vi "extract_pressure_SPT25.vi"(6 "name":string="AIN1", 8 "name_array":string[](array[string]), 9 "value_array":dbl[](array[numeric]), 11 "time":timestamp) -> (0 "P":dbl, 2 "V":dbl, 3 "waveform_array":waveform(dbl)[](array[waveform])=[{"t0"=timestamp(0 s since 1904-01-01), "dt"=1.0, "Y"=[]}, {"t0"=timestamp(3732035173.078092 s since 1904-01-01), "dt"=1.0, "Y"=[302.8589782714844], "attributes"=variant("NI_ChannelName"=variant(string "T1"))}])   [LabVIEW 2019]
panel:
  in  "V_max":dbl=10.0
  in  "V_min":dbl
  in  "P_max":dbl=30.0
  in  "P_min":dbl=-14.7
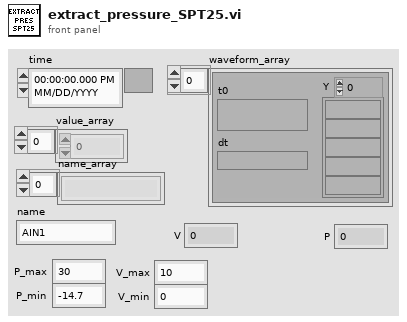
[diagram p1: front panel]
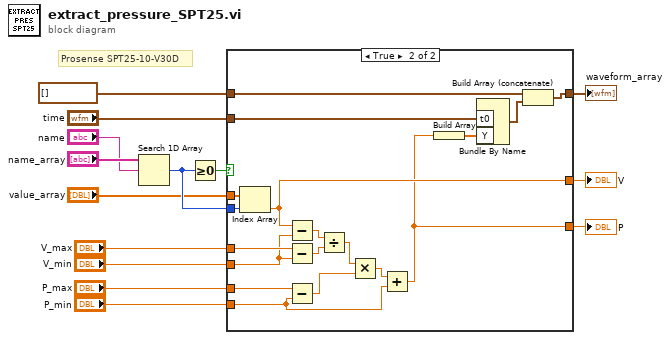
[diagram p0: block diagram]
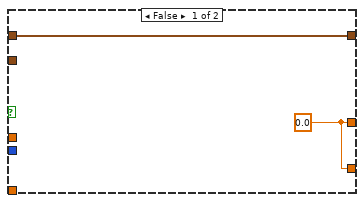
[diagram p2: hidden frame]
diagram:
  # "Prosense SPT25-10-V30D"
  n1 = Search 1D Array(1D array="name_array", element="name") -> (index of element=w11:i32)  [unwired: 1 in]
  n2 = Greater Or Equal To 0?(x=w11) -> (x >= 0?=w12:bool)
  n3 = case shown="True" w12 {
    tunnel: w11 -> [_ w34]
    tunnel: "value_array" -> [_ w33]
    tunnel: waveform(dbl)[] [] -> [w16 w32]
    tunnel: "time" -> [_ w31]
    tunnel: [w16 w30] -> w7
    tunnel: [w15 w17] -> w6
    tunnel: [w15 w25] -> w5
    tunnel: "P_min" -> [_ w18]
    tunnel: "P_max" -> [_ w22]
    tunnel: "V_max" -> [_ w27]
    tunnel: "V_min" -> [_ w26]
    frame False {
      w15 = 0.0 ("CJC (K)")
    }
    frame True {
      n4 = Index Array(array=w33, index=w34) -> (element=w25:dbl)
      n5 = Subtract(x=w25, y=w26) -> (x-y=w23:dbl)
      n6 = Subtract(x=w27, y=w26) -> (x-y=w24:dbl)
      n7 = Subtract(x=w22, y=w18) -> (x-y=w21:dbl)
      n8 = Divide(x=w23, y=w24) -> (x/y=w20:dbl)
      n9 = Multiply(x=w20, y=w21) -> (x*y=w19:dbl)
      n10 = Add(x=w19, y=w18) -> (x+y=w17:dbl)
      n11 = Build Array(w17) -> (w29:dbl[])
      n12 = Bundle By Name("t0"=w31, "Y"=w29) -> (w28:waveform(dbl))  [unwired: 1 in]
      n13 = Build Array (concatenate)(w32, w28) -> (w30:waveform(dbl)[])
    }
  }
  "waveform_array" <- w7
  "P" <- w6
  "V" <- w5
